vi "Vertex Logarithm Check.vi"(9 "Vertex Array In":sgl[](array[numeric]), 11 "Range Min":sgl) -> (1 "Vertex Array Out":sgl[](array[numeric]))   [LabVIEW 2020, in "3D Plot.lvclass"]
uses:
  <vilib>/Math Plots/3D Math Plots/3D Plot/3D Plot/3D Plot.lvclass
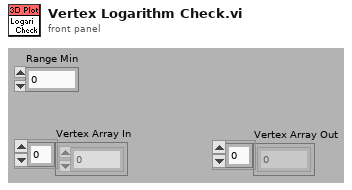
[diagram p1: front panel]
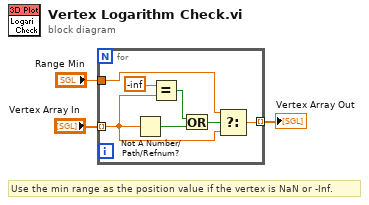
[diagram p0: block diagram]
diagram:
  # "Use the min range as the position value if the vertex is NaN or -Inf."
  n1 = for {
    tunnel: "Vertex Array In" -> [w4] mode=indexing
    tunnel: [w6] -> w3 mode=indexing
    tunnel: "Range Min" -> [w5]
    n2 = Not A Number/Path/Refnum?(number/path/refnum=w4) -> (NaN/Path/Refnum?=w9:bool)
    n3 = Equal?(x=sgl -inf, y=w4) -> (x = y?=w8:bool)
    n4 = Or(x=w8, y=w9) -> (x .or. y?=w7:bool)
    n5 = Select(t=w5, s=w7, f=w4) -> (s? t:f=w6:sgl)
  }
  "Vertex Array Out" <- w3
